vi "Get LoopTunnel Inside Terminal Wire Name.vi"(11 "Terminal in":refnum<vi>) -> (1 "InsideTerms[]":refnum<vi>[](array[refnum]), 2 "LoopTunnel inside wire names":string[](array[string]), 3 "LoopTunnel first inside wire name":string)   [LabVIEW 2018]
doc: "Returns name of wire connected to inside terminal of specified LoopTunnel. Every LoopTunnel has one output and more inside terminals.\nIn case that wire is not named, it returns name as 'wireUID_[wire uid]'."
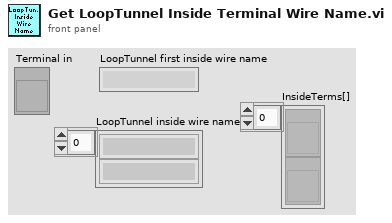
[diagram p1: front panel]
types:
  T1 = cluster{"wire labels":string[], "wire terminals datatypes":string[][]}
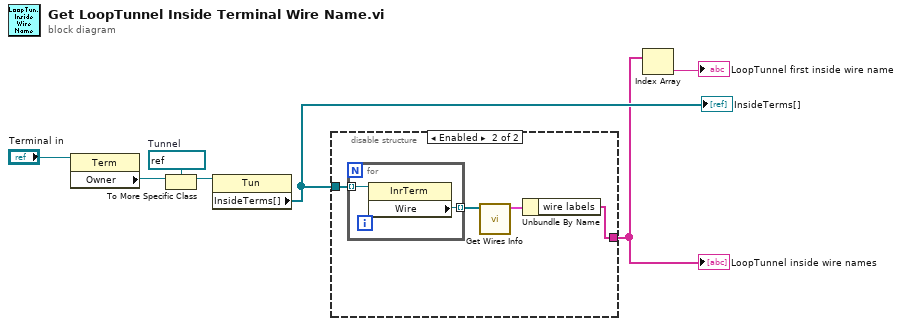
[diagram p0: block diagram]
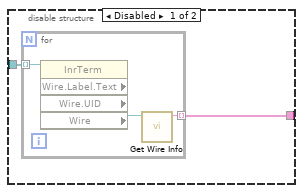
[diagram p2: hidden frame]
diagram:
  w2 = refnum<vi> refnum  # Tunnel
  n1 = property class="Term"(reference="Terminal in") -> ("Owner"=w5:refnum<vi>)  [unwired: 1 in, 2 out]
  n2 = To More Specific Class(target class=w2, reference=w5) -> (specific class reference=w1:refnum<vi>)  [unwired: 1 in, 1 out]
  n3 = property class="Tun"(reference=w1) -> ("InsideTerms[]"=w6:refnum<vi>[])  [unwired: 1 in, 2 out]
  "InsideTerms[]" <- w6
  n4 = disable-structure shown="Enabled" {
    disable-tunnel: w6 -> [w9 w16]
    disable-tunnel: [w8 w13] -> w4
    frame Disabled {
      n5 = for {
        tunnel: w9 -> [w10] mode=indexing
        tunnel: [w11] -> w8 mode=indexing
        n6 = property class="InrTerm" props=["Wire", "Label", "Text", "Wire", "UID", "Wire"](reference=w10) -> ("Wire"=w12:refnum<vi>)  [unwired: 1 in, 4 out]
        n7 = call "Get Wire Info.vi"("Wire"=w12) -> ("wire label"=w11:string)  [unwired: 9 in, 1 out]
      }
    }
    frame Enabled {
      n8 = for {
        tunnel: w16 -> [w18] mode=indexing
        tunnel: [w17] -> w15 mode=indexing
        n9 = property class="InrTerm"(reference=w18) -> ("Wire"=w17:refnum<vi>)  [unwired: 1 in, 2 out]
      }
      n10 = call "Get Wires Info.vi"("connected\nwires refs."=w15) -> ("wires info cluster"=w14:T1)  [unwired: 10 in]
      n11 = Unbundle By Name(w14) -> ("wire labels"=w13:string[])
    }
  }
  "LoopTunnel inside wire names" <- w4
  n12 = Index Array(array=w4) -> (element=→"LoopTunnel first inside wire name":string)  [unwired: 1 in]
